vi "Convert byte array.vi"(11 "Byte Array":u8[](array[numeric])) -> (0 "Hex String":string, 1 "Dot Hex String":string, 2 "Dot Decimal String":string, 3 "Double":dbl format="%.2f")   [LabVIEW 2021]
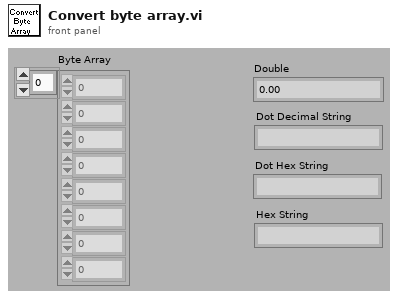
[diagram p1: front panel]
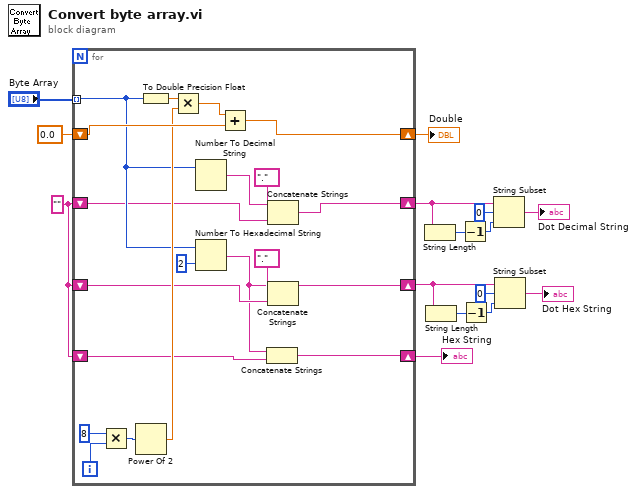
[diagram p0: block diagram]
diagram:
  w2 = ""
  n1 = for {
    tunnel: "Byte Array" -> [w27] mode=indexing
    shift-right: [w30] -> w14
    shift-left: 0.0 -> [w31]
    shift-right: [w26] -> w10
    shift-left: w2 -> [w23]
    shift-right: [w20] -> w4
    shift-left: w2 -> [w21]
    shift-right: [w18] -> w1
    shift-left: w2 -> [w17]
    i -> [w35]
    n2 = Multiply(x=8, y=w35) -> (x*y=w33:i32)
    n3 = Power Of 2(x=w33) -> (2^x=w29:dbl)
    n4 = To Double Precision Float(number=w27) -> (double precision float=w28:dbl)
    n5 = Multiply(x=w28, y=w29) -> (x*y=w32:dbl)
    n6 = Number To Decimal String(number=w27) -> (decimal integer string=w25:string)  [unwired: 1 in]
    n7 = Number To Hexadecimal String(1:i16 2 ("width (-)"), 2:w27) -> (0:w19:string)
    n8 = Add(x=w32, y=w31) -> (x+y=w30:dbl)
    n9 = Concatenate Strings(w19, w17) -> (w18:string)
    n10 = Concatenate Strings(w25, "." ("Substring"), w23) -> (w26:string)
    n11 = Concatenate Strings(w19, "." ("Substring"), w21) -> (w20:string)
  }
  "Double" <- w14
  "Hex String" <- w1
  n12 = String Length(string=w10) -> (length=w11:i32)
  n13 = String Length(string=w4) -> (length=w6:i32)
  n14 = Decrement(x=w11) -> (x-1=w12:i32)
  n15 = Decrement(x=w6) -> (x-1=w5:i32)
  n16 = String Subset(string=w10, offset (0)=0, length (rest)=w12) -> (substring=→"Dot Decimal String":string)
  n17 = String Subset(string=w4, offset (0)=0, length (rest)=w5) -> (substring=→"Dot Hex String":string)
